vi "Write Speed and Direction Speed Msg.vi"(3 "Use PWM?":bool, 4 "Offset":i32=200, 5 "Right Controller X Axis":i32, 6 "Left Controller Y Axis":i32) -> (0 "Left Motor":i16, 1 "Right Motor":i16, 2 "Speed UDP Message":string)   [LabVIEW 2015]
uses:
  <vilib>/gmath/NI_Gmath.lvlib
panel:
  out "Content length":i32
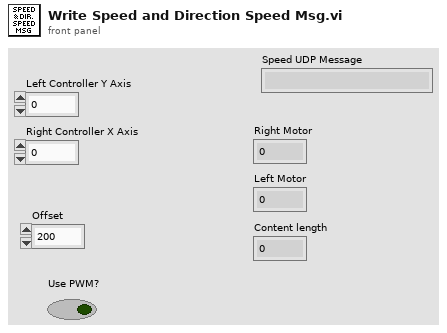
[diagram p1: front panel]
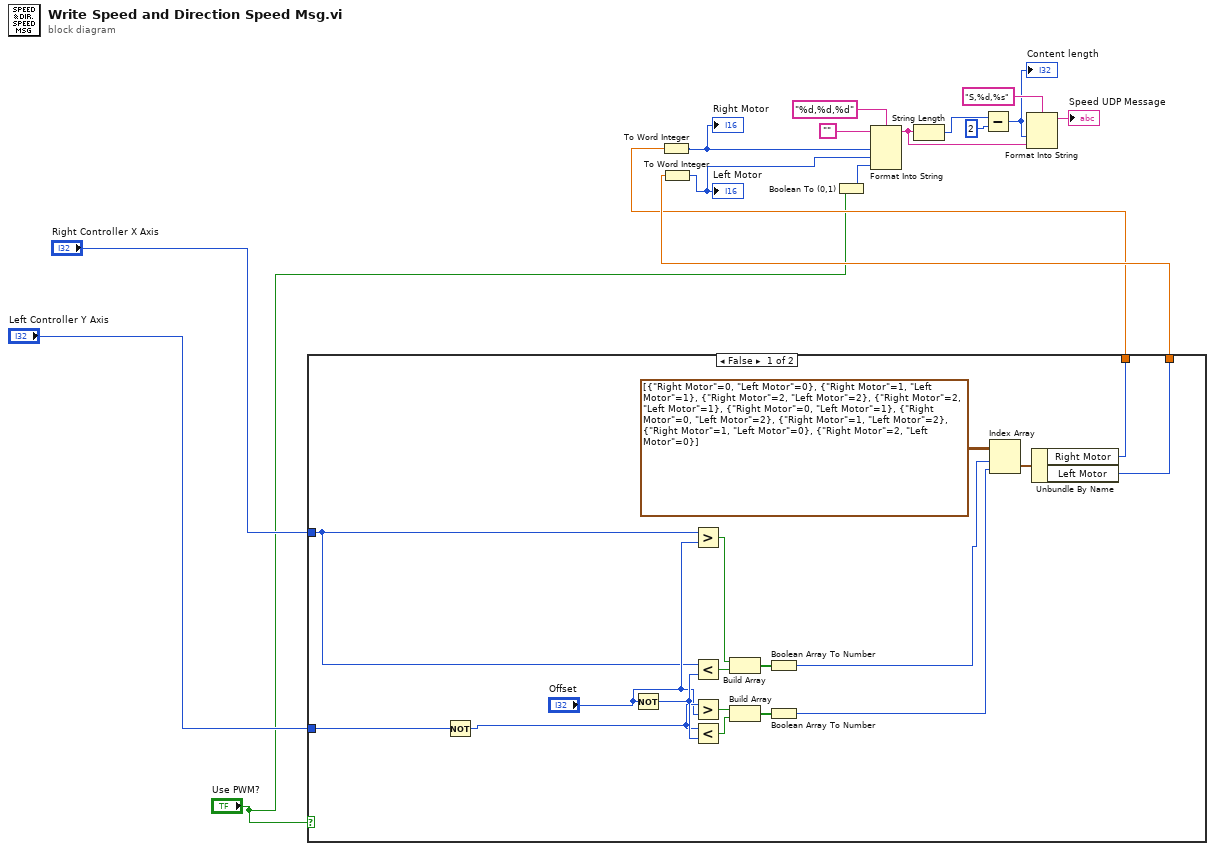
[diagram p0: block diagram]
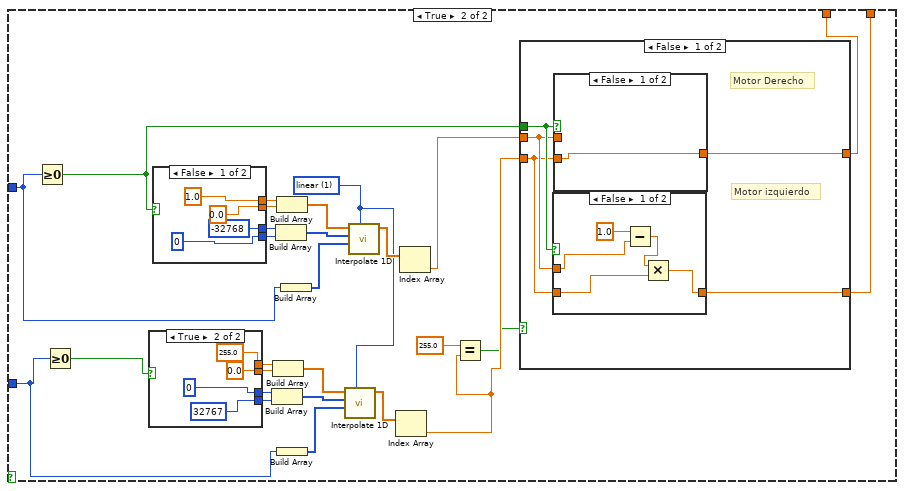
[diagram p2: hidden frame]
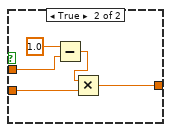
[diagram p4: hidden frame]
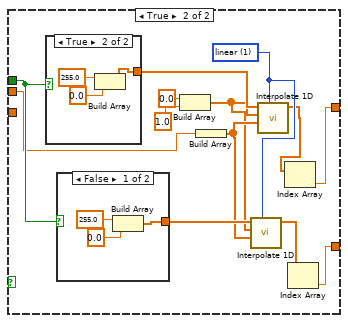
[diagram p5: hidden frame]
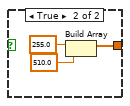
[diagram p6: hidden frame]
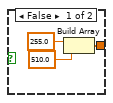
[diagram p7: hidden frame]
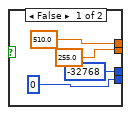
[diagram p8: hidden frame]
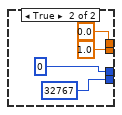
[diagram p9: hidden frame]
diagram:
  n1 = case shown="False" "Use PWM?" {
    tunnel: "Right Controller X Axis" -> [w17 w54]
    tunnel: "Left Controller Y Axis" -> [w26 w42]
    tunnel: [w19 w40] -> w3
    tunnel: [w18 w38] -> w6
    frame False {
      n2 = Not(x=w26) -> (.not. x?=w25:i32)
      n3 = Not(x="Offset") -> (.not. x?=w27:i32)
      n4 = Greater?(x=w17, y="Offset") -> (0:w29:bool)
      n5 = Less?(x=w17, y=w27) -> (x < y?=w30:bool)
      n6 = Greater?(x=w25, y="Offset") -> (0:w33:bool)
      n7 = Less?(x=w25, y=w27) -> (x < y?=w32:bool)
      n8 = Build Array(w29, w30) -> (w28:bool[])
      n9 = Build Array(w33, w32) -> (w31:bool[])
      n10 = Boolean Array To Number(Boolean array=w28) -> (number=w21:u32)
      n11 = Boolean Array To Number(Boolean array=w31) -> (number=w20:u32)
      n12 = Index Array(array=cluster{"Right Motor":i8, "Left Motor":i8}[][] [[{"Right Motor"=0, "Left Motor"=0}, {"Right Motor"=1, "Left Motor"=1}, {"Right Motor"=2, "Left Motor"=2}], [{"Right Motor"=2, "Left Motor"=1}, {"Right Motor"=0, "Left Motor"=1}, {"Right Motor"=0, "Left Motor"=2}], [{"Right Motor"=1, "Left Motor"=2}, {"Right Motor"=1, "Left Motor"=0}, {"Right Motor"=2, "Left Motor"=0}]], index (row)=w21, index (col)=w20) -> (element=w23:cluster{"Right Motor":i8, "Left Motor":i8})
      n13 = Unbundle By Name(w23) -> ("Right Motor"=w19:i8, "Left Motor"=w18:i8)
    }
    frame True {
      w37 = 1 items=["nearest", "linear", "spline", "cubic Hermite", "Lagrange"] ("method")
      n14 = Greater Or Equal To 0?(x=w54) -> (x >= 0?=w41:bool)
      n15 = Greater Or Equal To 0?(x=w42) -> (x >= 0?=w43:bool)
      n16 = case shown="True" w43 {
        tunnel: [i16 0 i16 32767 ("element")] -> w46
        tunnel: [i16 -32768 i16 0] -> w47
        tunnel: [255.0 ("element") 0.0 ("element")] -> w48
        tunnel: [510.0 ("element") 255.0 ("element")] -> w49
        frame False {
        }
        frame True {
        }
      }
      n17 = case shown="False" w41 {
        tunnel: [i16 0 i16 32767 ("element")] -> w58
        tunnel: [i16 -32768 i16 0] -> w57
        tunnel: [0.0 ("element") 1.0 ("element")] -> w56
        tunnel: [1.0 ("element") 0.0 ("element")] -> w55
        frame False {
        }
        frame True {
        }
      }
      n18 = Build Array(w47, w46) -> (w44:i16[])
      n19 = Build Array(w49, w48) -> (w45:dbl[])
      n20 = Build Array(w57, w58) -> (w60:i16[])
      n21 = Build Array(w55, w56) -> (w59:dbl[])
      n22 = Build Array(w42) -> (w50:i32[])
      n23 = Build Array(w54) -> (w53:i32[])
      n24 = call <vilib>:"Interpolate 1D.vi"("method"=w37, "xi"=w50, "X"=w44, "Y"=w45) -> ("yi"=w51:dbl[])  [unwired: 5 in, 2 out]
      n25 = call <vilib>:"Interpolate 1D.vi"("method"=w37, "xi"=w53, "X"=w60, "Y"=w59) -> ("yi"=w52:dbl[])  [unwired: 5 in, 2 out]
      n26 = Index Array(array=w51) -> (element=w35:dbl)  [unwired: 1 in]
      n27 = Index Array(array=w52) -> (element=w39:dbl)  [unwired: 1 in]
      n28 = Equal?(x=255.0, y=w35) -> (x = y?=w34:bool)
      n29 = case shown="False" w34 {
        tunnel: w41 -> [w65 w90]
        tunnel: [w64 w81] -> w40
        tunnel: w39 -> [w63 w86]
        tunnel: w35 -> [w62 _]
        tunnel: [w61 w80] -> w38
        frame False {
          # "Motor Derecho"
          # "Motor izquierdo"
          n30 = case shown="False" w65 {
            tunnel: w63 -> [w68 _]
            tunnel: w62 -> [w67 w71]
            tunnel: [w66 w71] -> w61
            frame False {
              n31 = Subtract(x=1.0, y=w68) -> (x-y=w70:dbl)
              n32 = Multiply(x=w70, y=w67) -> (x*y=w66:dbl)
            }
            frame True {
            }
          }
          n33 = case shown="False" w65 {
            tunnel: w62 -> [w72 w77]
            tunnel: w63 -> [_ w75]
            tunnel: [w72 w73] -> w64
            frame False {
            }
            frame True {
              n34 = Subtract(x=1.0, y=w75) -> (x-y=w74:dbl)
              n35 = Multiply(x=w74, y=w77) -> (x*y=w73:dbl)
            }
          }
        }
        frame True {
          w82 = 1 items=["nearest", "linear", "spline", "cubic Hermite", "Lagrange"] ("method")
          n36 = case shown="True" w90 {
            tunnel: [w97 w100] -> w88
            frame False {
              n37 = Build Array(255.0 ("element"), 510.0 ("element")) -> (w97:dbl[])
            }
            frame True {
              n38 = Build Array(255.0 ("element"), 0.0 ("element")) -> (w100:dbl[])
            }
          }
          n39 = case shown="False" w90 {
            tunnel: [w92 w94] -> w85
            frame False {
              n40 = Build Array(255.0 ("element"), 0.0 ("element")) -> (w92:dbl[])
            }
            frame True {
              n41 = Build Array(255.0 ("element"), 510.0 ("element")) -> (w94:dbl[])
            }
          }
          n42 = Build Array(0.0 ("element"), 1.0 ("element")) -> (w83:dbl[])
          n43 = Build Array(w86) -> (w84:dbl[])
          n44 = call <vilib>:"Interpolate 1D.vi"("method"=w82, "xi"=w84, "X"=w83, "Y"=w85) -> ("yi"=w78:dbl[])  [unwired: 5 in, 2 out]
          n45 = call <vilib>:"Interpolate 1D.vi"("method"=w82, "xi"=w84, "X"=w83, "Y"=w88) -> ("yi"=w79:dbl[])  [unwired: 5 in, 2 out]
          n46 = Index Array(array=w79) -> (element=w81:dbl)  [unwired: 1 in]
          n47 = Index Array(array=w78) -> (element=w80:dbl)  [unwired: 1 in]
        }
      }
    }
  }
  n48 = To Word Integer(number=w3) -> (16bit integer=w4:i16)
  "Right Motor" <- w4
  n49 = To Word Integer(number=w6) -> (16bit integer=w5:i16)
  "Left Motor" <- w5
  n50 = Boolean To (0,1)(Boolean="Use PWM?") -> (0, 1=w2:i16)
  n51 = Format Into String(format string="%d,%d,%d", initial string="", w4, w5, w2) -> (resulting string=w14:string)  [unwired: 1 in, 1 out]
  n52 = String Length(string=w14) -> (length=w11:i32)
  n53 = Subtract(x=w11, y=2) -> (x-y=w9:i32)
  "Content length" <- w9
  n54 = Format Into String(format string="S,%d,%s", w9, w14) -> (resulting string=→"Speed UDP Message":string)  [unwired: 2 in, 1 out]
